vi "TestCurrent.vi"() -> ()   [LabVIEW 2011]
panel:
  in  "stop 8":bool
  in  "stop 7":bool
  in  "stop 6":bool
  in  "stop 5":bool
  in  "stop 4":bool
  in  "stop 3":bool
  in  "stop 2":bool
  in  "stop":bool
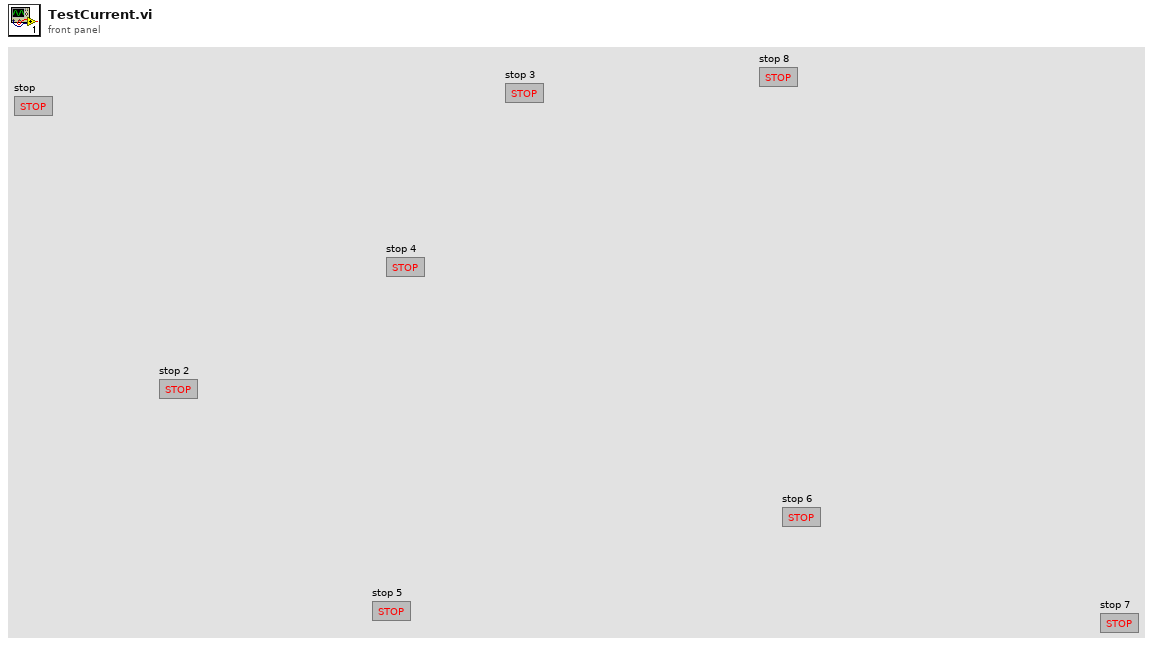
[diagram p1: front panel]
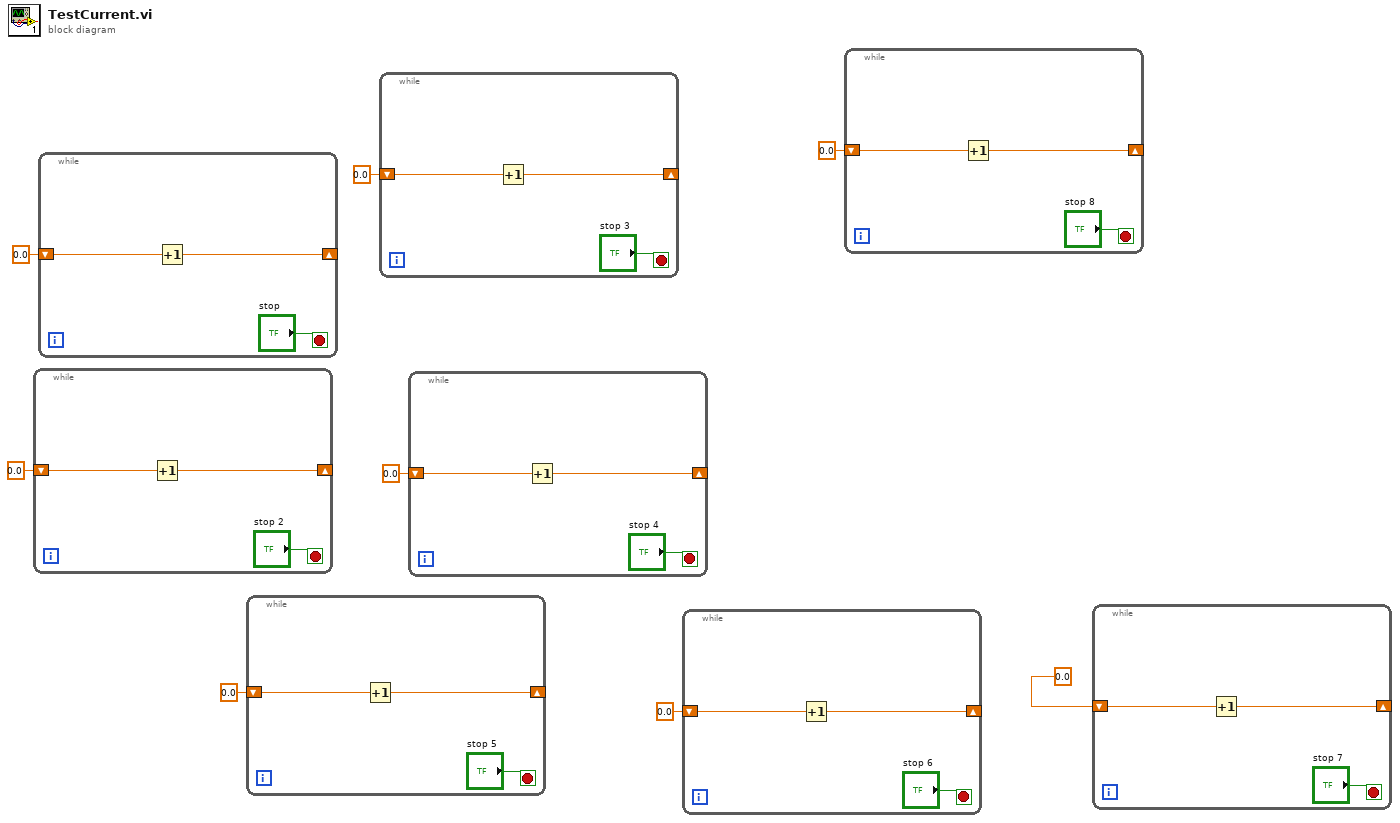
[diagram p0: block diagram]
diagram:
  n1 = while {
    shift-right: [w11] -> _
    shift-left: 0.0 -> [w10]
    stop <- "stop 2" stop-if-true
    n2 = Increment(x=w10) -> (x+1=w11:dbl)
  }
  n3 = while {
    shift-right: [w14] -> _
    shift-left: 0.0 -> [w13]
    stop <- "stop" stop-if-true
    n4 = Increment(x=w13) -> (x+1=w14:dbl)
  }
  n5 = while {
    shift-right: [w17] -> _
    shift-left: 0.0 -> [w16]
    stop <- "stop 5" stop-if-true
    n6 = Increment(x=w16) -> (x+1=w17:dbl)
  }
  n7 = while {
    shift-right: [w20] -> _
    shift-left: 0.0 -> [w19]
    stop <- "stop 3" stop-if-true
    n8 = Increment(x=w19) -> (x+1=w20:dbl)
  }
  n9 = while {
    shift-right: [w23] -> _
    shift-left: 0.0 -> [w22]
    stop <- "stop 4" stop-if-true
    n10 = Increment(x=w22) -> (x+1=w23:dbl)
  }
  n11 = while {
    shift-right: [w26] -> _
    shift-left: 0.0 -> [w25]
    stop <- "stop 6" stop-if-true
    n12 = Increment(x=w25) -> (x+1=w26:dbl)
  }
  n13 = while {
    shift-right: [w29] -> _
    shift-left: 0.0 -> [w28]
    stop <- "stop 8" stop-if-true
    n14 = Increment(x=w28) -> (x+1=w29:dbl)
  }
  n15 = while {
    shift-right: [w32] -> _
    shift-left: 0.0 -> [w31]
    stop <- "stop 7" stop-if-true
    n16 = Increment(x=w31) -> (x+1=w32:dbl)
  }
